vi "Post-Install Custom Action.vi"() -> (0 "error out":errorcluster)   [LabVIEW 2021]
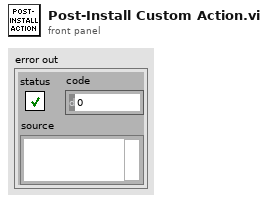
[diagram p1: front panel]
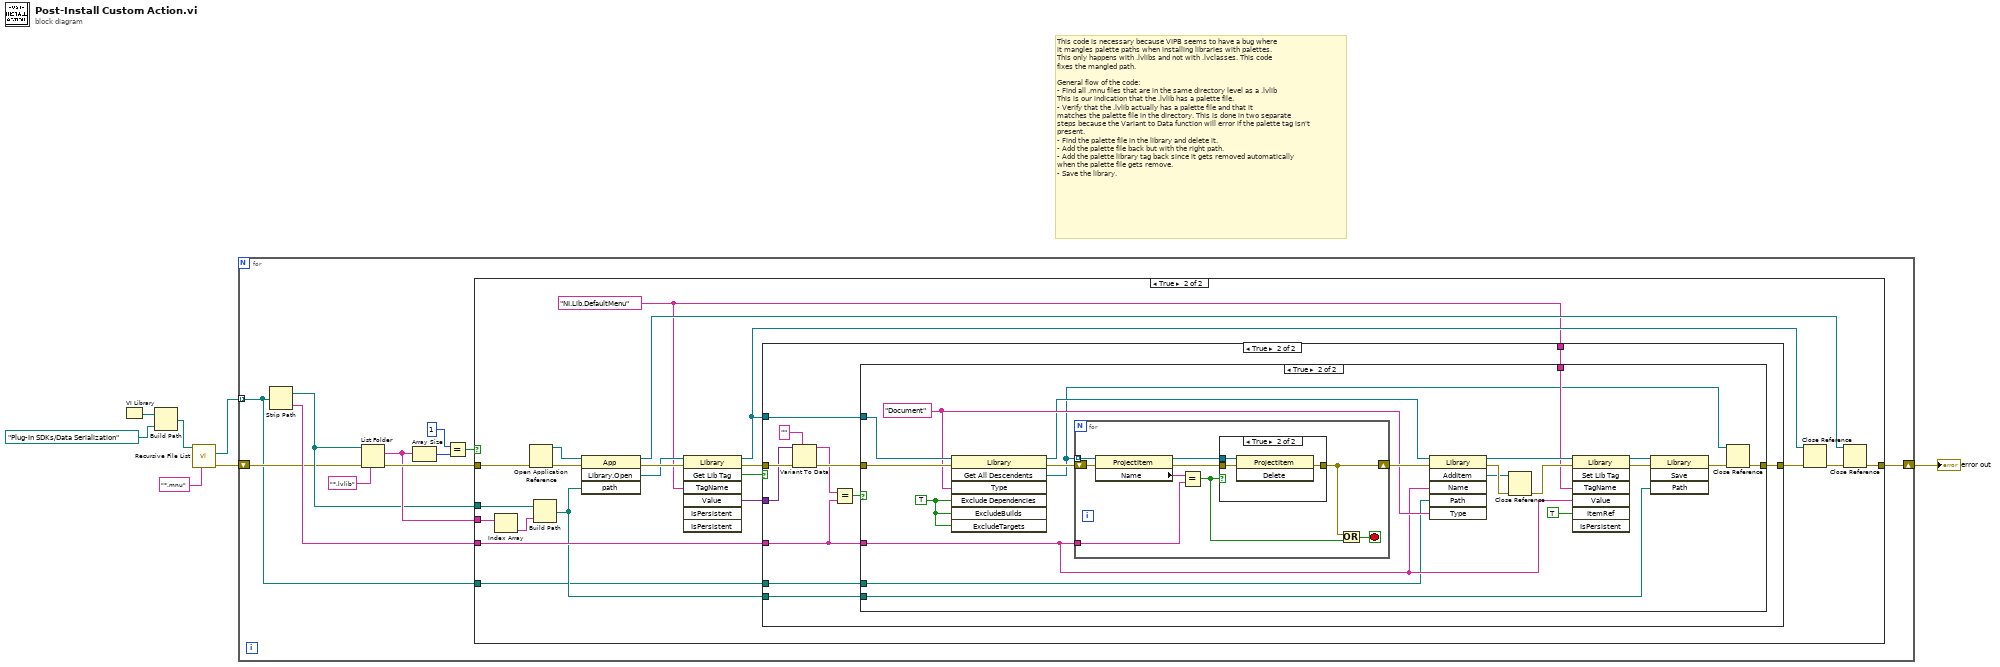
[diagram p0: block diagram]
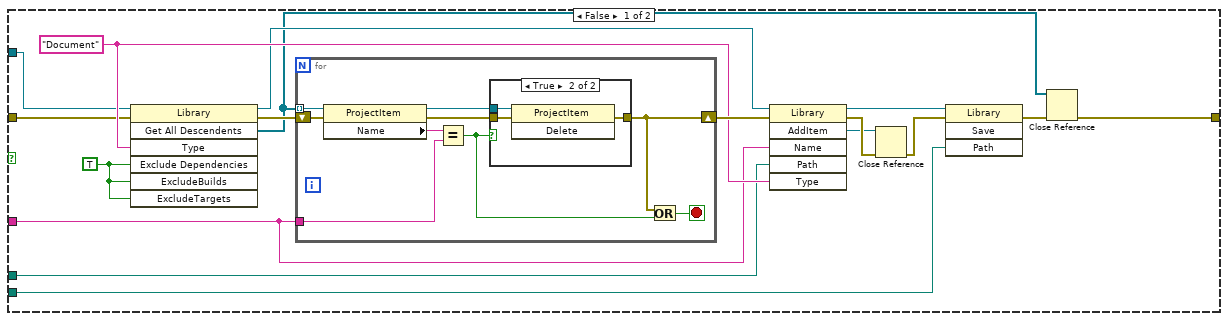
[diagram p4: hidden frame]
diagram:
  # "This code is necessary because VIPB seems to have a bug where\nit mangles palette paths when installing libraries with palettes.\nThis only happens with .lvlibs and not with .lvclasses. This code\nfixes the mangled path.\n\nGeneral flow of the code:\n- Find all .mnu files that are in the same directory level as a .lvlib\nThis is our indication that the .lvlib has a palette file.\n- Verify that the .lvlib actually has a palette file and that it\nmatches the palette file in the directory. This is done in two separate\nsteps because the Variant to Data function will error if the palette tag isn't\npresent.\n- Find the palette file in the library and delete it.\n- Add the palette file back but with the right path.\n- Add the palette library tag back since it gets removed automatically\nwhen the palette file gets remove.\n- Save the library."
  n1 = VI Library() -> (path=w5:path)
  n2 = Build Path(base path=w5, name or relative path=path "Plug-In SDKs/Data Serialization") -> (appended path=w6:path)
  n3 = call <vilib>:"Recursive File List.vi"("pattern"="*.mnu", "Folder Path"=w6) -> ("error out"=w2:errorcluster, "All Files in Dir"=w1:path[])  [unwired: 5 in, 3 out]
  n4 = for {
    shift-right: [w10] -> w7
    shift-left: w2 -> [w9]
    tunnel: w1 -> [w8] mode=indexing
    n5 = Strip Path(path=w8) -> (stripped path=w12:path, name=w16:string)
    n6 = List Folder(path=w12, pattern="*.lvlib", error in=w9) -> (filenames=w14:string[], error out=w15:errorcluster)  [unwired: 1 in, 2 out]
    n7 = Array Size(array=w14) -> (size(s)=w18:i32)
    n8 = Equal?(x=1, y=w18) -> (x = y?=w17:bool)
    n9 = case shown="True" w17 {
      tunnel: w15 -> [w19 w36]
      tunnel: w14 -> [_ w39]
      tunnel: w16 -> [_ w31]
      tunnel: w12 -> [_ w27]
      tunnel: [w19 w21] -> w10
      tunnel: w8 -> [_ w20]
      frame False {
      }
      frame True {
        w23 = "NI.Lib.DefaultMenu" ("Tag Name")
        n10 = Index Array(array=w39) -> (element=w26:string)  [unwired: 1 in]
        n11 = Open Application Reference(8:w36) -> (0:w38:errorcluster, 3:w37:refnum<vi>)  [unwired: 3 in]
        n12 = Build Path(base path=w27, name or relative path=w26) -> (appended path=w25:path)
        n13 = invoke class="App" method="Library.Open"(reference=w37, error in=w38, "path"=w25) -> (reference out=w28:refnum<vi>, error out=w35:errorcluster, "Open Library"=w32:refnum<vi>)  [unwired: 1 in, 1 out]
        n14 = invoke class="Library" method="Get Lib Tag"(reference=w32, error in=w35, "TagName"=w23) -> (reference out=w29:refnum<vi>, error out=w33:errorcluster, "GetTag"=w24:bool, "Value"=w34:variant)  [unwired: 4 in, 3 out]
        n15 = case shown="True" w24 {
          tunnel: w34 -> [_ w48]
          tunnel: w33 -> [w40 w49]
          tunnel: [w40 w52] -> w30
          tunnel: w29 -> [_ w51]
          tunnel: w25 -> [_ w50]
          tunnel: w31 -> [_ w44]
          tunnel: w23 -> [_ w42]
          tunnel: w20 -> [_ w41]
          frame False {
          }
          frame True {
            n16 = Variant To Data(error in=w49, type="", Variant=w48) -> (data=w45:string, error out=w47:errorcluster)
            n17 = Equal?(x=w45, y=w44) -> (x = y?=w43:bool)
            n18 = case shown="True" w43 {
              tunnel: [w53 w92] -> w52
              tunnel: w51 -> [w57 w103]
              tunnel: w50 -> [w54 w98]
              tunnel: w47 -> [w58 w97]
              tunnel: w44 -> [w56 w84]
              tunnel: w42 -> [_ w89]
              tunnel: w41 -> [w55 w83]
              frame False {
                w63 = "Document" ("Type")
                w61 = TRUE ("ExcludeDependencies")
                n19 = invoke class="Library" method="Get All Descendents"(reference=w57, error in=w58, "Type"=w63, "Exclude Dependencies"=w61, "ExcludeBuilds"=w61, "ExcludeTargets"=w61) -> (reference out=w60:refnum<vi>, error out=w69:errorcluster, "All Descendents"=w59:refnum<vi>[])  [unwired: 1 in, 4 out]
                n20 = for {
                  tunnel: w59 -> [w78] mode=indexing
                  shift-right: [w72] -> w68
                  shift-left: w69 -> [w74]
                  tunnel: w56 -> [w73]
                  stop <- w70 stop-if-true
                  n21 = property class="ProjectItem"(reference=w78, error in=w74) -> (reference out=w76:refnum<vi>, error out=w75:errorcluster, "Name"=w77:string)
                  n22 = Equal?(x=w77, y=w73) -> (x = y?=w71:bool)
                  n23 = case shown="True" w71 {
                    tunnel: w76 -> [_ w82]
                    tunnel: w75 -> [w79 w80]
                    tunnel: [w79 w81] -> w72
                    frame False {
                    }
                    frame True {
                      n24 = invoke class="ProjectItem" method="Delete"(reference=w82, error in=w80) -> (error out=w81:errorcluster)  [unwired: 1 in, 2 out]
                    }
                  }
                  n25 = Or(x=w72, y=w71) -> (x .or. y?=w70:bool)
                }
                n26 = invoke class="Library" method="AddItem"(reference=w60, error in=w68, "Name"=w56, "Path"=w55, "Type"=w63) -> (reference out=w62:refnum<vi>, error out=w66:errorcluster, "AddItem"=w65:refnum<vi>)  [unwired: 1 in, 3 out]
                n27 = Close Reference(reference=w65, error in (no error)=w66) -> (error out=w64:errorcluster)
                n28 = invoke class="Library" method="Save"(reference=w62, error in=w64, "Path"=w54) -> (error out=w67:errorcluster)  [unwired: 1 in, 3 out]
                n29 = Close Reference(reference=w59, error in (no error)=w67) -> (error out=w53:errorcluster)
              }
              frame True {
                w91 = "Document" ("Type")
                w87 = TRUE ("ExcludeDependencies")
                n30 = invoke class="Library" method="Get All Descendents"(reference=w103, error in=w97, "Type"=w91, "Exclude Dependencies"=w87, "ExcludeBuilds"=w87, "ExcludeTargets"=w87) -> (reference out=w86:refnum<vi>, error out=w102:errorcluster, "All Descendents"=w85:refnum<vi>[])  [unwired: 1 in, 4 out]
                n31 = for {
                  tunnel: w85 -> [w112] mode=indexing
                  shift-right: [w106] -> w101
                  shift-left: w102 -> [w108]
                  tunnel: w84 -> [w107]
                  stop <- w104 stop-if-true
                  n32 = property class="ProjectItem"(reference=w112, error in=w108) -> (reference out=w110:refnum<vi>, error out=w109:errorcluster, "Name"=w111:string)
                  n33 = Equal?(x=w111, y=w107) -> (x = y?=w105:bool)
                  n34 = case shown="True" w105 {
                    tunnel: w110 -> [_ w116]
                    tunnel: w109 -> [w113 w114]
                    tunnel: [w113 w115] -> w106
                    frame False {
                    }
                    frame True {
                      n35 = invoke class="ProjectItem" method="Delete"(reference=w116, error in=w114) -> (error out=w115:errorcluster)  [unwired: 1 in, 2 out]
                    }
                  }
                  n36 = Or(x=w106, y=w105) -> (x .or. y?=w104:bool)
                }
                n37 = invoke class="Library" method="AddItem"(reference=w86, error in=w101, "Name"=w84, "Path"=w83, "Type"=w91) -> (reference out=w90:refnum<vi>, error out=w95:errorcluster, "AddItem"=w94:refnum<vi>)  [unwired: 1 in, 3 out]
                n38 = Close Reference(reference=w94, error in (no error)=w95) -> (error out=w93:errorcluster)
                n39 = invoke class="Library" method="Set Lib Tag"(reference=w90, error in=w93, "TagName"=w89, "Value"=w84, "ItemRef"=TRUE ("Is Persistent")) -> (reference out=w100:refnum<vi>, error out=w99:errorcluster)  [unwired: 2 in, 5 out]
                n40 = invoke class="Library" method="Save"(reference=w100, error in=w99, "Path"=w98) -> (error out=w96:errorcluster)  [unwired: 1 in, 3 out]
                n41 = Close Reference(reference=w85, error in (no error)=w96) -> (error out=w92:errorcluster)
              }
            }
          }
        }
        n42 = Close Reference(reference=w29, error in (no error)=w30) -> (error out=w22:errorcluster)
        n43 = Close Reference(reference=w28, error in (no error)=w22) -> (error out=w21:errorcluster)
      }
    }
  }
  "error out" <- w7
